vi "Potting Data - Address Pads.vi"(10 "Address Pads Selection":cluster{"Top":bool, "Bottom":bool}, 11 "Address Pads Data":T2) -> (3 "Potting Lines":T1[](array[typedef]))   [LabVIEW 2011]
uses:
  Shared Components/Utils/Type Definitions/Multi-Fiducial Image.ctl
  Shared Components/Vec3d Class/Vec3d Class.lvclass
  Shared Components/Utils/Type Definitions/Physical Image.ctl
  <vilib>/vision/Image Controls.llb/IMAQ Image.ctl
  Shared Components/Utils/Type Definitions/Fiducial with Source.ctl
  Shared Components/Utils/Type Definitions/3d Line.ctl
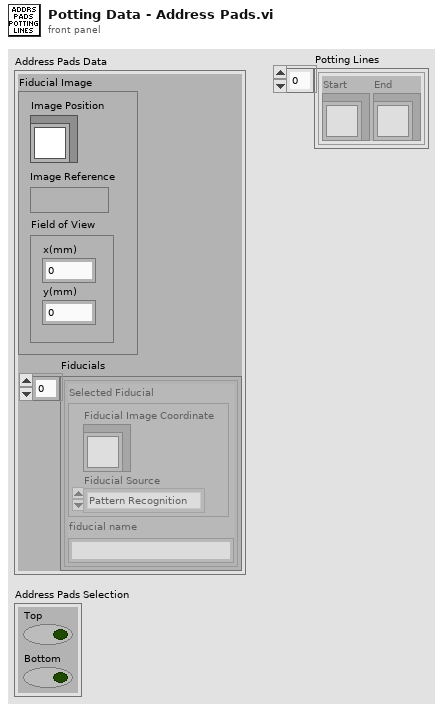
[diagram p1: front panel]
types:
  T1 = typedef "3d Line.ctl" = cluster{"Start":refnum<class "Vec3d Class.lvclass">, "End":refnum<class "Vec3d Class.lvclass">}
  T2 = typedef "Multi-Fiducial Image.ctl" = cluster{"Fiducial Image":T3, "Fiducials":cluster{"Selected Fiducial":T5, "fiducial name":string}[]}
  T3 = typedef "Physical Image.ctl" = cluster{"Image Position":refnum<class "Vec3d Class.lvclass">, "Image Reference":T4, "Field of View":cluster{"x(mm)":dbl, "y(mm)":dbl}}
  T4 = typedef "IMAQ Image.ctl" = refnum<image>
  T5 = typedef "Fiducial with Source.ctl" = cluster{"Fiducial Image Coordinate":refnum<class "Vec3d Class.lvclass">, "Fiducial Source":enum16{"Pattern Recognition", "User", "Error", "Default"}}
  T6 = cluster{"Selected Fiducial":T5, "fiducial name":string}[]
  T7 = cluster{"Selected Fiducial":T5, "fiducial name":string}
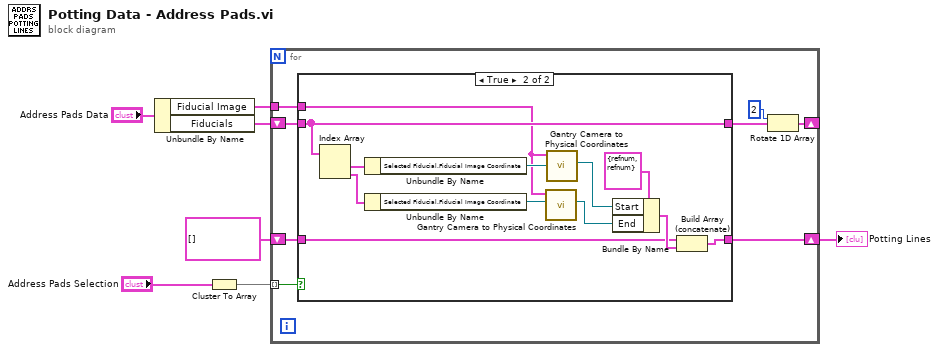
[diagram p0: block diagram]
diagram:
  n1 = Unbundle By Name("Address Pads Data") -> ("Fiducial Image"=w1:T3, "Fiducials"=w5:T6)
  n2 = Cluster To Array(cluster="Address Pads Selection") -> (array=w6:bool[])
  n3 = for {
    tunnel: w6 -> [w15] mode=indexing
    shift-right: [w9] -> _
    shift-left: w5 -> [w14]
    shift-right: [w12] -> w3
    shift-left: T1[] [] -> [w13]
    tunnel: w1 -> [w8]
    n4 = case shown="True" w15 {
      tunnel: w14 -> [w16 w29]
      tunnel: [w16 w29] -> w10
      tunnel: w13 -> [w17 w24]
      tunnel: [w17 w23] -> w12
      tunnel: w8 -> [_ w21]
      frame False {
      }
      frame True {
        n5 = Index Array(array=w29) -> (element #1=w27:T7, element #2=w28:T7)  [unwired: 2 in]
        n6 = Unbundle By Name(w27) -> ("Selected Fiducial.Fiducial Image Coordinate"=w22:refnum<class "Vec3d Class.lvclass">)
        n7 = Unbundle By Name(w28) -> ("Selected Fiducial.Fiducial Image Coordinate"=w20:refnum<class "Vec3d Class.lvclass">)
        n8 = call "Gantry Camera to Physical Coordinates.vi"("Image Coordinate"=w20, "Physical Image"=w21) -> ("Global Coordinate"=w18:refnum<class "Vec3d Class.lvclass">)  [unwired: 7 in, 2 out]
        n9 = call "Gantry Camera to Physical Coordinates.vi"("Image Coordinate"=w22, "Physical Image"=w21) -> ("Global Coordinate"=w19:refnum<class "Vec3d Class.lvclass">)  [unwired: 7 in, 2 out]
        n10 = Bundle By Name(cluster=T1 {"Start"=refnum, "End"=refnum} ("3D Line"), "Start"=w19, "End"=w18) -> (w25:T1)
        n11 = Build Array (concatenate)(w24, w25) -> (w23:T1[])
      }
    }
    n12 = Rotate 1D Array(1:w10, 2:2 ("n")) -> (0:w9:T6)
  }
  "Potting Lines" <- w3
